vi "Read terminals.vi"(8 "error in (no error)":errorcluster, 11 "BlockDiagram in":refnum<class "AbstractDiagram.lvclass">) -> (0 "error out":errorcluster, 2 "terminals":refnum<class "Terminal.lvclass">[](array[class]), 3 "BlockDiagram out":refnum<class "AbstractDiagram.lvclass">)   [LabVIEW 2023, in "TLC_Scripto.lvlib" / "AbstractDiagram.lvclass"]
uses:
  AbstractDiagram.lvclass
  AbstractDiagram.lvclass/AbstractDiagram.ctl
  Terminal/Terminal.lvclass
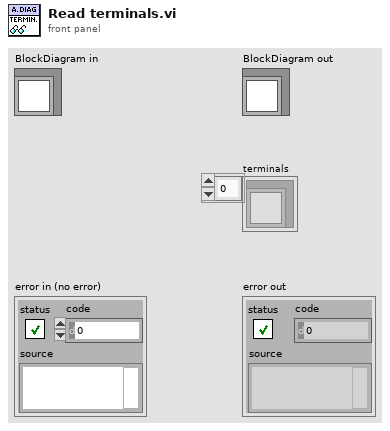
[diagram p1: front panel]
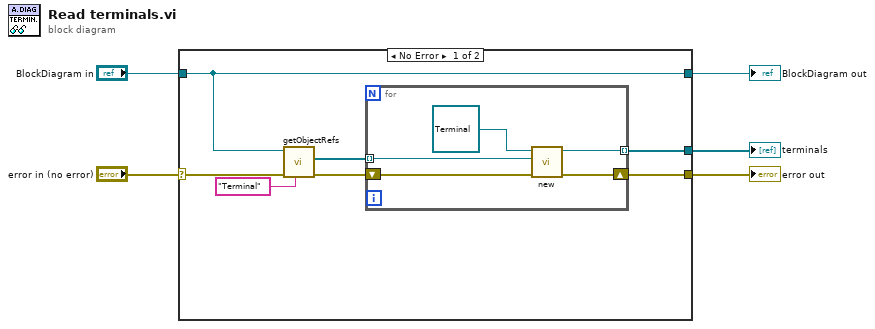
[diagram p0: block diagram]
diagram:
  n1 = case shown="No Error" "error in (no error)" {
    selector: "error in (no error)" -> [w8 w19]
    tunnel: [w7 w19] -> w4
    tunnel: [w9 w18] -> w2
    tunnel: "BlockDiagram in" -> [w9 w18]
    tunnel: [w6 _] -> w1
    frame No Error {
      n2 = call "getObjectRefs.vi"("type(ClassName)"="Terminal" ("Class Name"), "error in (no error)"=w8, "BlockDiagram in"=w9) -> ("error out"=w10:errorcluster, "refs"=w11:refnum<vi>[])  [unwired: 6 in, 1 out]
      n3 = for {
        tunnel: w11 -> [w17] mode=indexing
        shift-right: [w15] -> w7
        shift-left: w10 -> [w16]
        tunnel: [w14] -> w6 mode=indexing
        n4 = call-dynamic "new.vi"("Error In"=w16, "ref"=w17, "Generic In"=refnum<class "Terminal.lvclass"> refnum ("TLC_Scripto.lvlib:Terminal")) -> ("Error Out"=w15:errorcluster, "Generic Out"=w14:refnum<class "Terminal.lvclass">)  [unwired: 7 in]
      }
    }
    frame Error {
    }
  }
  "error out" <- w4
  "BlockDiagram out" <- w2
  "terminals" <- w1
